vi "GV_SetToolbar.vi"(8 "error in (no error)":errorcluster, 11 "Gviewer in":refnum<class "Gviewer.lvclass">) -> (0 "error out":errorcluster, 3 "Gviewer out":refnum<class "Gviewer.lvclass">)   [LabVIEW 2020, in "Gviewer.lvclass"]
doc: "Set the Size and Position of the GViewer toolbar"
uses:
  Gviewer.lvclass
  <vilib>/Utility/miscctls.llb/LVPositionTypeDef.ctl
  <vilib>/Utility/miscctls.llb/LVBoundsTypeDef.ctl
  Gviewer.lvclass/Gviewer.ctl
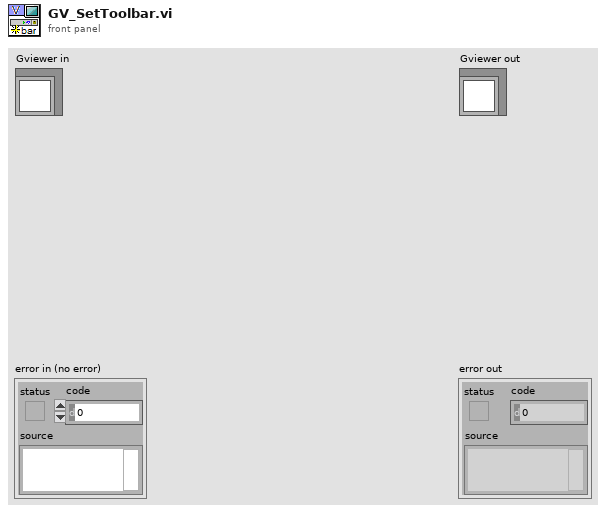
[diagram p1: front panel]
types:
  T1 = typedef "LVBoundsTypeDef.ctl" = cluster{"Width":u32, "Height":u32}
  T2 = typedef "LVPositionTypeDef.ctl" = cluster{"Left":i32, "Top":i32}
  T3 = cluster{"left":i16, "top":i16, "right":i16, "bottom":i16}
  T4 = typedef "ToolBarAppearance.ctl" = enum16{"Bare", "Native", "Gradient"}
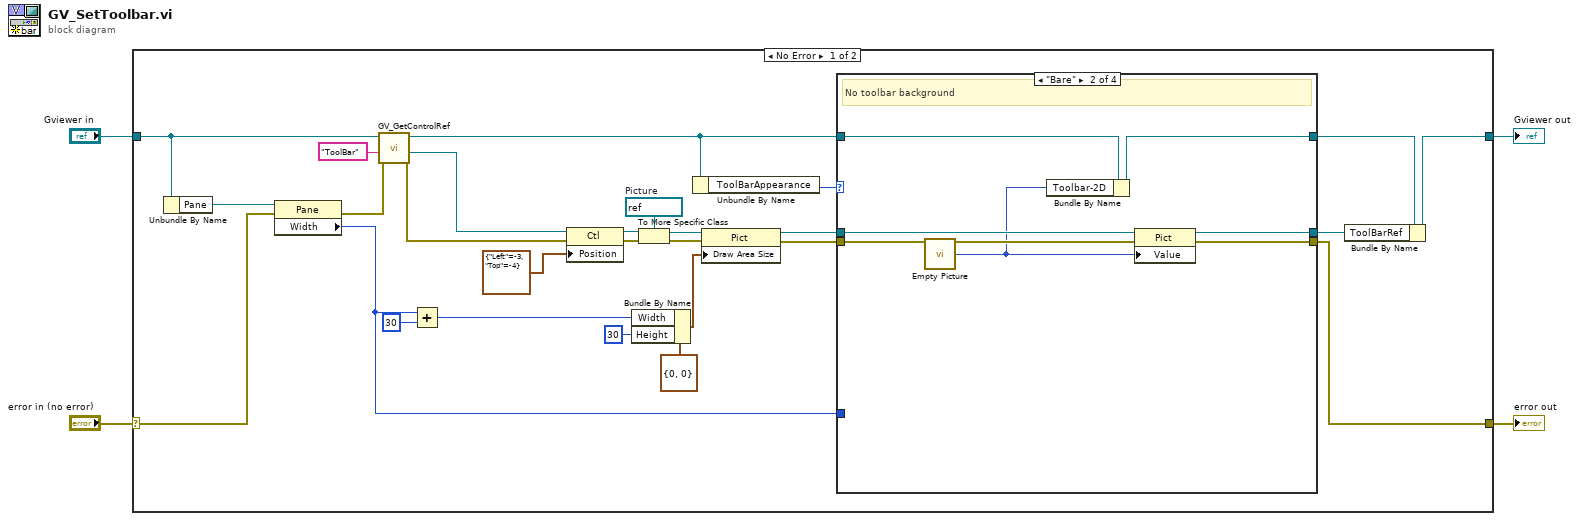
[diagram p0: block diagram]
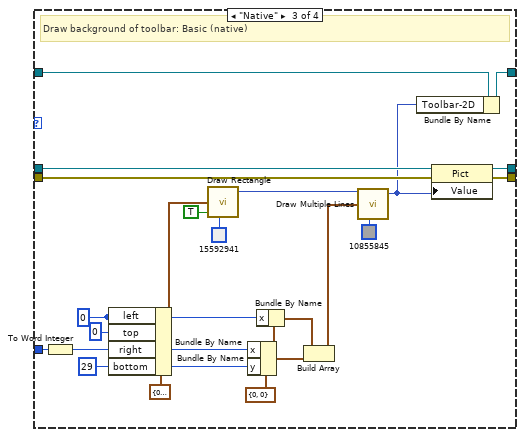
[diagram p3: hidden frame]
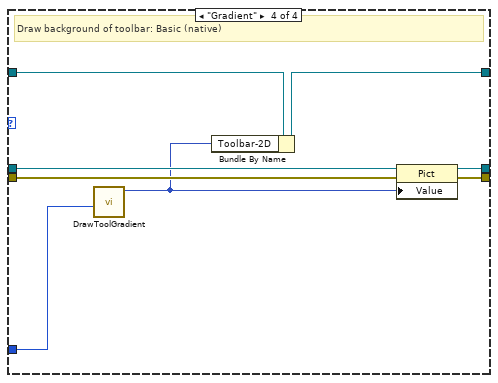
[diagram p4: hidden frame]
diagram:
  n1 = case shown="No Error" "error in (no error)" {
    selector: "error in (no error)" -> [w16 w73]
    tunnel: [w10 w73] -> w3
    tunnel: [w5 w72] -> w1
    tunnel: "Gviewer in" -> [w15 w72]
    frame No Error {
      w26 = refnum<vi> refnum  # Picture
      n2 = Unbundle By Name(w15) -> ("Pane"=w14:refnum<vi>)
      n3 = property class="Pane"(reference=w14, error in=w16) -> (error out=w19:errorcluster, "Width"=w8:u32)  [unwired: 1 out]
      n4 = call "GV_GetControlRef.vi"("error in (no error)"=w19, "CNT name"="ToolBar", "Gviewer in"=w15) -> ("error out"=w29:errorcluster, "Reference"=w30:refnum<vi>, "Gviewer out"=w12:refnum<class "Gviewer.lvclass">)  [unwired: 6 in]
      n5 = Add(x=w8, y=u32 30) -> (x+y=w17:u32)
      n6 = property class="Ctl"(reference=w30, error in=w29, "Position"=T2 {"Left"=-3, "Top"=-4}) -> (reference out=w27:refnum<vi>, error out=w25:errorcluster)
      n7 = Bundle By Name(cluster=T1 {"Width"=0, "Height"=0} ("Draw Area Size"), "Width"=w17, "Height"=u32 30) -> (w21:T1)
      n8 = To More Specific Class(target class=w26, reference=w27, error in=w25) -> (specific class reference=w24:refnum<vi>, error out=w23:errorcluster)
      n9 = Unbundle By Name(w12) -> ("ToolBarAppearance"=w13:T4)
      n10 = property class="Pict"(reference=w24, error in=w23, "Draw Area Size"=w21) -> (reference out=w9:refnum<vi>, error out=w11:errorcluster)
      n11 = case shown="\"Bare\"" w13 {
        tunnel: w12 -> [w34 w37 w44 w66]
        tunnel: [w34 w38 w45 w67] -> w6
        tunnel: w11 -> [w33 w40 w62 w70]
        tunnel: [w33 w39 w61 w69] -> w10
        tunnel: w9 -> [w32 w41 w63 w71]
        tunnel: w8 -> [_ _ w58 w68]
        tunnel: [w32 w35 w42 w64] -> w7
        frame Default {
        }
        frame "Bare" {
          # "No toolbar background"
          n12 = call "Empty Picture"() -> ("empty picture"=w36:picture)
          n13 = Bundle By Name(cluster=w37, "Toolbar-2D"=w36) -> (w38:refnum<class "Gviewer.lvclass">)
          n14 = property class="Pict"(reference=w41, error in=w40, "Value"=w36) -> (reference out=w35:refnum<vi>, error out=w39:errorcluster)
        }
        frame "Native" {
          w47 = i16 29 ("bottom")
          w46 = i16 0 ("bottom")
          # "Draw background of toolbar: Basic (native)"
          n15 = To Word Integer(number=w58) -> (16bit integer=w51:i16)
          n16 = Bundle By Name(cluster=T3 {"left"=0, "top"=0, "right"=0, "bottom"=0} ("rect"), "left"=w46, "top"=i16 0 ("bottom"), "right"=w51, "bottom"=w47) -> (w57:T3)
          n17 = call <vilib>:"Draw Rectangle.vi"("rect"=w57, "fill?(F)"=TRUE, "color(black)"=u32 15592941) -> ("new picture"=w54:picture)  [unwired: 6 in]
          n18 = Bundle By Name(cluster=cluster{"x":i16, "y":i16} {"x"=0, "y"=0}, "x"=w51, "y"=w47) -> (w49:cluster{"x":i16, "y":i16})
          n19 = Bundle By Name(cluster=w49, "x"=w46) -> (w50:cluster{"x":i16, "y":i16})
          n20 = Build Array(w50, w49) -> (w48:cluster{"x":i16, "y":i16}[])
          n21 = call <vilib>:"Draw Multiple Lines.vi"("picture"=w54, "line endpoints"=w48, "color(black)"=u32 10855845) -> ("new picture"=w43:picture)  [unwired: 6 in]
          n22 = Bundle By Name(cluster=w44, "Toolbar-2D"=w43) -> (w45:refnum<class "Gviewer.lvclass">)
          n23 = property class="Pict"(reference=w63, error in=w62, "Value"=w43) -> (reference out=w42:refnum<vi>, error out=w61:errorcluster)
        }
        frame "Gradient" {
          # "Draw background of toolbar: Basic (native)"
          n24 = call "DrawToolGradient.vi"("Width"=w68) -> ("Background"=w65:picture)  [unwired: 10 in]
          n25 = Bundle By Name(cluster=w66, "Toolbar-2D"=w65) -> (w67:refnum<class "Gviewer.lvclass">)
          n26 = property class="Pict"(reference=w71, error in=w70, "Value"=w65) -> (reference out=w64:refnum<vi>, error out=w69:errorcluster)
        }
      }
      n27 = Bundle By Name(cluster=w6, "ToolBarRef"=w7) -> (w5:refnum<class "Gviewer.lvclass">)
    }
    frame Error {
    }
  }
  "error out" <- w3
  "Gviewer out" <- w1
